vi "LAC Cmd120_Disp setting.vi"(6 "R/W (F:Read)":bool, 7 "timeout(ms)":u32, 8 "error in":errorcluster, 9 "Items":T1, 11 "VISA name in":refnum<visa-resource-name>) -> (0 "error out":errorcluster, 1 "readout":string, 3 "VISA name out":refnum<visa-resource-name>)   [LabVIEW 8.6]
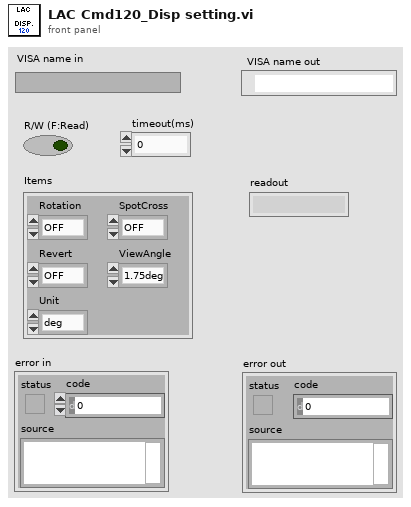
[diagram p1: front panel]
types:
  T1 = cluster{"Rotation":enum16{"OFF", "90deg CCW", "90deg CC"}, "Revert":enum16{"OFF", "X On", "Y On", "XY On"}, "Unit":enum16{"deg", "min+sec", "mrad"}, "SpotCross":enum16{"OFF", "ON"}, "ViewAngle":enum16{"1.75deg", "1.00deg", "0.50deg", "0.25deg"}}
  T2 = enum16{"1.75deg", "1.00deg", "0.50deg", "0.25deg"}
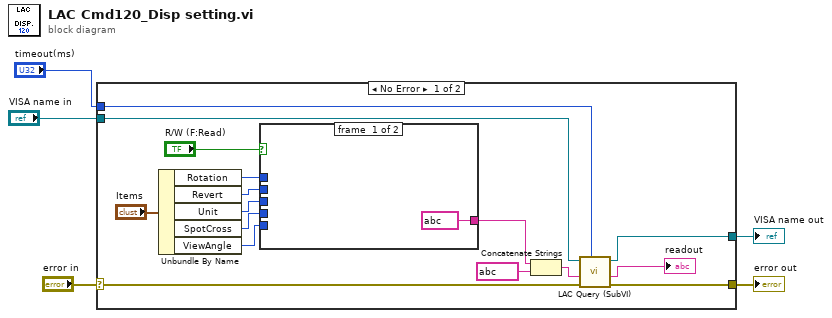
[diagram p0: block diagram]
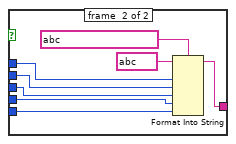
[diagram p2: hidden frame]
diagram:
  n1 = case shown="No Error" "error in" {
    selector: "error in" -> [w17 w32]
    tunnel: "VISA name in" -> [w19 w31]
    tunnel: [w21 w31] -> w4
    tunnel: [w20 w32] -> w3
    tunnel: "timeout(ms)" -> [w18 _]
    frame #0 {
      n2 = Unbundle By Name("Items") -> ("Rotation"=w6:enum16{"OFF", "90deg CCW", "90deg CC"}, "Revert"=w7:enum16{"OFF", "X On", "Y On", "XY On"}, "Unit"=w8:enum16{"deg", "min+sec", "mrad"}, "SpotCross"=w9:enum16{"OFF", "ON"}, "ViewAngle"=w10:T2)
      n3 = case shown="True" "R/W (F:Read)" {
        tunnel: [string ? ("string") w29] -> w14
        tunnel: w7 -> [_ w28]
        tunnel: w6 -> [_ w27]
        tunnel: w8 -> [_ w25]
        tunnel: w9 -> [_ w24]
        tunnel: w10 -> [_ w23]
        frame #0 {
        }
        frame #1 {
          n4 = Format Into String(format string=string ?, initial string=string ? ("string"), w27, w28, w25, w24, w23) -> (resulting string=w29:string)  [unwired: 1 in, 1 out]
        }
      }
      n5 = Concatenate Strings(w14, string ? ("write buffer")) -> (w15:string)
      n6 = call "LAC Query (SubVI).vi"("timeout(ms)"=w18, "error in"=w17, "Command"=w15, "VISA name in"=w19) -> ("error out"=w20:errorcluster, "read buffer"=→"readout":string, "VISA name out"=w21:refnum<visa-resource-name>)  [unwired: 5 in]
    }
    frame #1 {
    }
  }
  "VISA name out" <- w4
  "error out" <- w3
